vi "S2C_ExeScriptResultUpdate.vi"(5 "LastMeas?":bool, 7 "LastTest?":bool, 8 "Error In":errorcluster, 9 "StepSettings":string, 10 "MeasName":string, 11 "Measurement":string) -> (0 "Error Out":errorcluster, 1 "Time":string, 2 "MeasOut":string, 3 "Result":T1)   [LabVIEW 2015]
doc: "Determines the result for the currently executing line item, and updates the measurement and result in the data array."
uses:
  Controls/S2C_ResultStatus.ctl
  Globals/S2C_Globals.vi
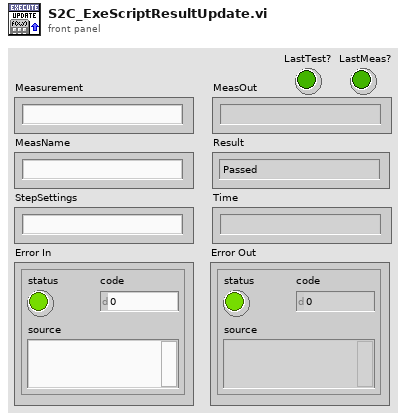
[diagram p1: front panel]
types:
  T1 = typedef "S2C_ResultStatus.ctl" = enum16{"Passed", "Failed", "Logged", "Aborted", "Error", "Testing...", "Paused", "No Record"}
  T2 = cluster{"Step Type":string, "High Limit":string, "High Limit Comparison":string, "Low Limit":string, "Low Limit Comparison":string, "Units":string, "Log Step":string, "Record Step":string}
  T3 = cluster{"MeasName":string, "MeasDateTime":string, "Comment":string, "MeasType":string, "MeasValue":string, "TargetValue":string, "HL Comp":string, "HighLimit":string, "LL Comp":string, "LowLimit":string, "Units":string, "MeasStatus":string}
  T4 = cluster{"MeasName":string, "MeasDateTime":string, "MeasStatus":string, "MeasClientID":string, "IS_MeasID":string, "MeasType":string, "MeasValue":string, "LL":string, "LL Comp":string, "HL":string, "HL Comp":string, "Units":string, "MeasMeta":string}
  T5 = cluster{"EventStatus":string, "TestStatus":string, "MeasStatus":string}
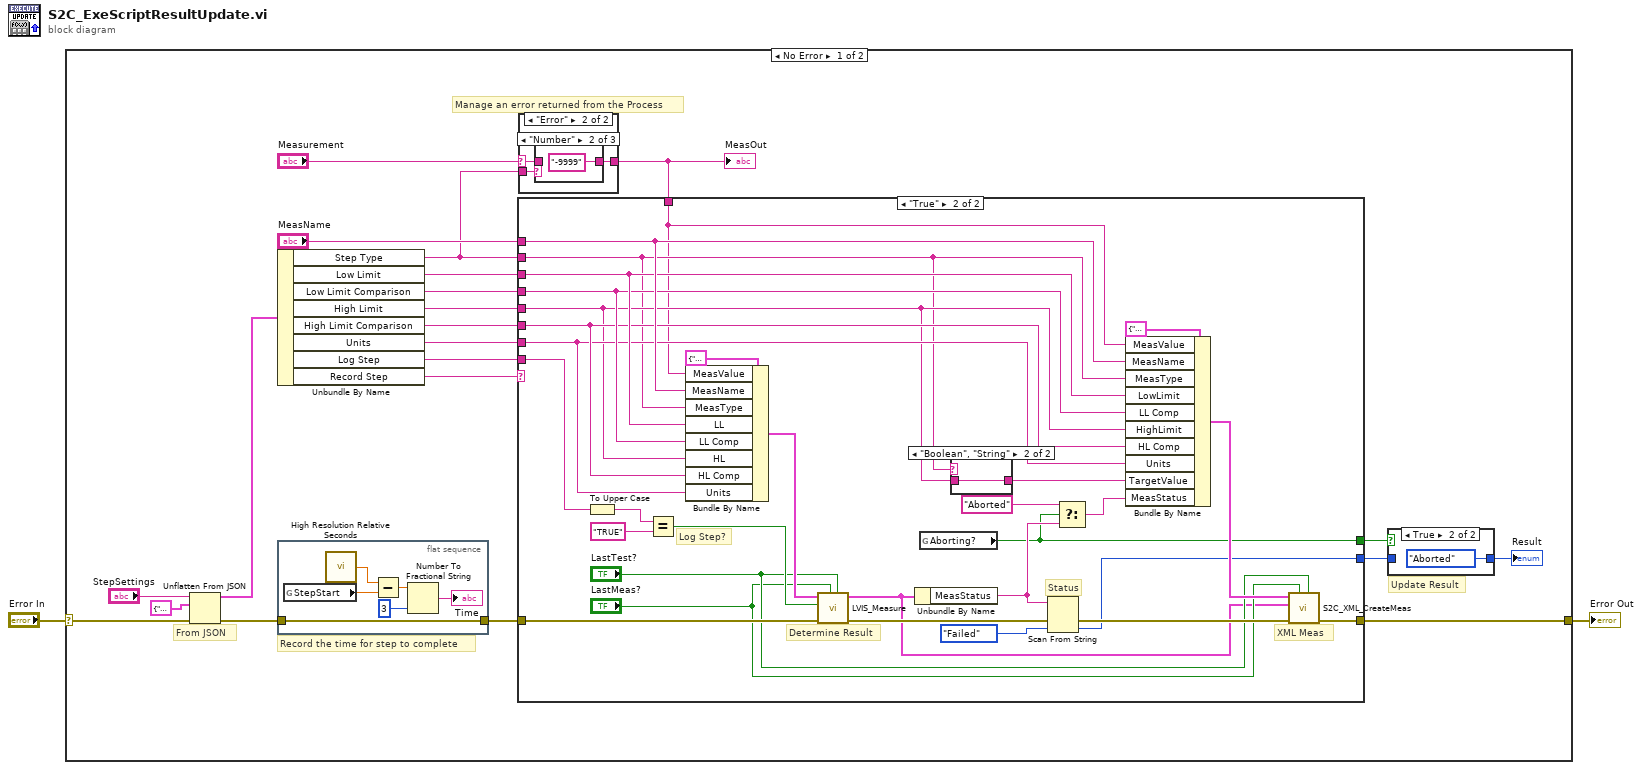
[diagram p0: block diagram]
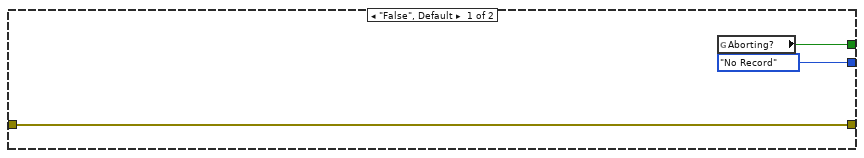
[diagram p2: hidden frame]
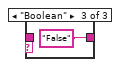
[diagram p7: hidden frame]
diagram:
  n1 = case shown="No Error" "Error In" {
    selector: "Error In" -> [w21 w73]
    tunnel: [w8 w73] -> w1
    frame No Error {
      # "Record the time for step to complete"
      # "Update Result"
      # "Manage an error returned from the Process"
      # "From JSON"
      n2 = Unflatten From JSON(JSON string="StepSettings", type and defaults=T2 {"Step Type"="", "High Limit"="", "High Limit Comparison"="", "Low Limit"="", "Low Limit Comparison"="", "Units"="", "Log Step"="", "Record Step"=""}, error in (no error)=w21) -> (value=w23:T2, error out=w4:errorcluster)  [unwired: 4 in]
      n3 = Unbundle By Name(w23) -> ("Step Type"=w12:string, "Low Limit"=w18:string, "Low Limit Comparison"=w17:string, "High Limit"=w14:string, "High Limit Comparison"=w16:string, "Units"=w15:string, "Log Step"=w22:string, "Record Step"=w5:string)
      n4 = flat-sequence {
        tunnel: w4 -> [w29]
        tunnel: [w29] -> w3
        frame #0 {
          n5 = global read "S2C_Globals.vi" "StepStart"() -> (w25:dbl)
          n6 = call <vilib>:"High Resolution Relative Seconds.vi"() -> ("relative seconds"=w24:dbl)
          n7 = Subtract(x=w24, y=w25) -> (x-y=w27:dbl)
          n8 = Number To Fractional String(number=w27, precision (6)=i16 3) -> (F-format string=→"Time":string)  [unwired: 2 in]
        }
      }
      n9 = case shown="\"Error\"" "Measurement" {
        selector: "Measurement" -> [w66 w67]
        tunnel: w12 -> [_ w69]
        tunnel: [w66 w68] -> w6
        frame "Other", Default {
        }
        frame "Error" {
          n10 = case shown="\"Number\"" w69 {
            tunnel: [w70 "-9999" "False"] -> w68
            tunnel: w67 -> [w70 _ _]
            frame "String", Default {
            }
            frame "Number" {
            }
            frame "Boolean" {
            }
          }
        }
      }
      "MeasOut" <- w6
      n11 = case shown="\"True\"" w5 {
        tunnel: w3 -> [w32 w60]
        tunnel: w22 -> [_ w58]
        tunnel: "MeasName" -> [_ w53]
        tunnel: w18 -> [_ w52]
        tunnel: w17 -> [_ w51]
        tunnel: w16 -> [_ w50]
        tunnel: w15 -> [_ w49]
        tunnel: w14 -> [_ w47]
        tunnel: w12 -> [_ w42]
        tunnel: [w31 w41] -> w10
        tunnel: [S2C_ResultStatus."No Record" ("Status") w39] -> w9
        tunnel: [w32 w38] -> w8
        tunnel: w6 -> [_ w37]
        frame "False", Default {
          n12 = global read "S2C_Globals.vi" "Aborting?"() -> (w31:bool)
        }
        frame "True" {
          # "Log Step?"
          # "XML Meas"
          # "Status"
          # "Determine Result"
          n13 = To Upper Case(1:w58) -> (0:w57:string)
          n14 = Equal?(x=w57, y="TRUE") -> (x = y?=w55:bool)
          n15 = Bundle By Name(cluster=T4 {"MeasName"="", "MeasDateTime"="", "MeasStatus"="", "MeasClientID"="", "IS_MeasID"="", "MeasType"="", "MeasValue"="", "LL"="", "LL Comp"="", "HL"="", "HL Comp"="", "Units"="", "MeasMeta"=""} ("MeasInfo"), "MeasValue"=w37, "MeasName"=w53, "MeasType"=w42, "LL"=w52, "LL Comp"=w51, "HL"=w47, "HL Comp"=w50, "Units"=w49) -> (w61:T4)
          n16 = call "LVIS_Measure.vi"("LastEventMeas?"="LastTest?", "LastTestMeas?"="LastMeas?", "Error In"=w60, "Log Step?"=w55, "MeasInfo"=w61) -> ("Error Out"=w34:errorcluster, "Status"=w33:T5)  [unwired: 5 in]
          n17 = Unbundle By Name(w33) -> ("MeasStatus"=w44:string)
          n18 = global read "S2C_Globals.vi" "Aborting?"() -> (w41:bool)
          n19 = case shown="\"Boolean\", \"String\"" w42 {
            tunnel: w47 -> [_ w63]
            tunnel: [_ w63] -> w46
            frame "Other", Default {
            }
            frame "Boolean", "String" {
            }
          }
          n20 = Scan From String(input string=w44, error in=w34, default 1=S2C_ResultStatus."Failed" ("Status")) -> (error out=w40:errorcluster, output 1=w39:T1)  [unwired: 2 in, 2 out]
          n21 = Select(t="Aborted", s=w41, f=w44) -> (s? t:f=w43:string)
          n22 = Bundle By Name(cluster=T3 {"MeasName"="", "MeasDateTime"="", "Comment"="", "MeasType"="", "MeasValue"="", "TargetValue"="", "HL Comp"="", "HighLimit"="", "LL Comp"="", "LowLimit"="", "Units"="", "MeasStatus"=""} ("MeasData"), "MeasValue"=w37, "MeasName"=w53, "MeasType"=w42, "LowLimit"=w52, "LL Comp"=w51, "HighLimit"=w47, "HL Comp"=w50, "Units"=w49, "TargetValue"=w46, "MeasStatus"=w43) -> (w48:T3)
          n23 = call "S2C_XML_CreateMeas.vi"("LastTest?"="LastTest?", "LastMeas?"="LastMeas?", "Error In"=w40, "Result"=w33, "MeasData"=w48) -> ("Error Out"=w38:errorcluster)  [unwired: 6 in]
        }
      }
      n24 = case shown="True" w10 {
        tunnel: w9 -> [w64 _]
        tunnel: [w64 S2C_ResultStatus."Aborted" ("Status")] -> w7
        frame False {
        }
        frame True {
        }
      }
      "Result" <- w7
    }
    frame Error {
    }
  }
  "Error Out" <- w1
